vi "AIM664 VL Receive.vi"() -> ()   [LabVIEW 2020]
uses:
  AIM664LV.lvlib
panel:
  out "error out":errorcluster
  out "MsgErrorCount 2":u32
  out "MsgCount 2":u32
  out "MsgErrorCount":u32
  out "MsgCount":u32
  out "ReadBuffer 2":u8[](array[numeric])
  out "MsgRead 2":u32
  out "ReadBuffer":u8[](array[numeric])
  out "MsgRead":u32
  in  "RxModeControlIn":T1={"ReceiveMode"=1, "DefaultPayloadMode"=0, "DefaultCronoMode"=1, "GlbMonBufferSizeIn"=0, "RerosDefaultOutputPortmap"=0} {"ReceiveMode" items=["FDX_RX_CHRONO", "FDX_RX_VL"]; "DefaultPayloadMode" items=["FDX_PAYLOAD_FULL", "FDX_PAYLOAD_IP_EXT", "FDX_PAYLOAD_IP", "FDX_PAYLOAD_MAC"]; "DefaultCronoMode" items=["cFDX_RX_DEFAULT_ENA_CNT", "FDX_RX_DEFAULT_MON_ENA_ALL", "FDX_RX_DEFAULT_MON_ENA_GOOD"]}
  in  "PortMap":u32
  in  "While-Loop-Stop":bool
  in  "UdpPort2Description":T2={"PortType"=0, "UdpSrc"=2, "IpSrc"=167846145, "VlId"=10, "IpDst"=3772776458, "UdpDst"=2, "SubVlId"=0, "UdpNumBufMessages"=1, "UdpMaxMessageSize"=128, "UdpSamplingRate"=16} {"IpDst" format="%x"; "IpSrc" format="%x"; "PortType" items=["FDX_UDP_SAMPLING", "FDX_UDP_QUEUING", "FDX_UDP_RX_SAP", "FDX_UDP_TX_SAP"]}
  in  "UdpPort1Description":T2={"PortType"=0, "UdpSrc"=1, "IpSrc"=167846145, "VlId"=10, "IpDst"=3772776458, "UdpDst"=1, "SubVlId"=0, "UdpNumBufMessages"=1, "UdpMaxMessageSize"=128, "UdpSamplingRate"=32} {"IpDst" format="%x"; "IpSrc" format="%x"; "PortType" items=["FDX_UDP_SAMPLING", "FDX_UDP_QUEUING", "FDX_UDP_RX_SAP", "FDX_UDP_TX_SAP"]}
  in  "VLControl":T3={"VLId"=10, "VLRange"=1, "EnableMode"=4, "PayloadMode"=0, "TCBIndex"=0, "VerificationMode"=0, "Bag"=8, "Jitter"=1, "MaxFrameLength"=1024, "MaxSkew"=5000, "VLBufSize"=0, "FilterMode"=0, "FilterPosition"=0, "Padding"=0, "FilterMask"=0, "FilterData"=0, "MinFrameLength"=0} {"EnableMode" items=["FDX_RX_VL_DIS "=0, "FDX_RX_VL_ENA_STAT"=1, "FDX_RX_VL_ENA_CNT "=2, "FDX_RX_VL_ENA_MON_ALL"=3, "FDX_RX_VL_ENA_MON_GOOD"=7, "FDX_RX_VL_ENA_EXT"=4]; "PayloadMode" items=["FDX_PAYLOAD_FULL", "FDX_PAYLOAD_IP_EXT", "FDX_PAYLOAD_IP", "FDX_PAYLOAD_MAC"]; "VerificationMode" items=["FDX_RX_VL_CHECK_ENA_DEFAULT"=65535, "FDX_RX_VL_CHECK_REDMAM"=16, "DX_RX_VL_CHECK_TRAFIC"=8, "FDX_RX_VL_CHECK_FRAMESIZE"=4, "FDX_RX_VL_CHECK_SNINTEG"=2, "FDX_RX_VL_CHECK_INVPAC"=1, "FDX_RX_VL_CHECK_DISA"=0]; "FilterMode" items=["FDX_RX_VL_FLT_DIS", "FDX_RX_VL_FLT_ENA ", "FDX_RX_VL_FLT_ENA_INV"]}
  out "ResourceInfo 2":T4 {"PortMode" items=[" FDX_SINGLE", "FDX_REDUNDANT"]}
  out "ResourceInfo":T4 {"PortMode" items=[" FDX_SINGLE", "FDX_REDUNDANT"]}
  in  "Input Cluster":T5={"SrvName"="local", "ClHostName"="local", "ClUser"="Brett", "ClApplication"="Test", "ClApplicationVersion"="V01.00", "ResourceID"=2, "Privileges"=4294967295} {"Privileges" items=["PRIVILEGES_ADMIN"=4294967295]}
  in  "Input Cluster":T6={"SrvName"="local", "ResourceID"=1, "ResourceType"=0} {"ResourceType" items=["Board", "Port"]}
  out "Output Cluster 2":T7={"ResourceID"=1, "ResourceType"=0, "ResourceInfo"="AMC-FDX-2", "StructId"=0}
  in  "ServerRElement":u32=1
  in  "Input Cluster":T6={"SrvName"="local", "ResourceID"=2, "ResourceType"=1} {"ResourceType" items=["Board", "Port"]}
  out "Output Cluster":T7={"ResourceID"=2, "ResourceType"=1, "ResourceInfo"="Port1", "StructId"=0}
  in  "ServerRElement":u32=2
  out "NuOfResources":u32=3
  in  "SrvName":string="local"
  out "NuOfServers":u32=1
  # "ARINC 664 Receive data through a Virtual Link (VL)"
  # "Overview: Configure the board to write UDP blocks into a Port.\nRequirement: At least one AIM ARINC-664 board with installed AIM ARINC 664 BSP.\nRestrictions: None.\nInstruction:\n1. Run the VI.\n2. Verify the results in the indicators."
  # "Rx Port"
  # "FdxRxControlCvi (Stop Rx)"
  # "FdxLogoutCvi"
  # "Rx Port"
  # "Main UDP Read While-Loop"
  # "FdxInitCvi"
  # "CountServerResourcesCvi"
  # "GetServerResourcesCvi"
  # "FdxLoginCvi"
  # "FdxCmdRxPortInit"
  # "FdxCmdRxModeControl"
  # "FdxCmdVLRxControl"
  # "UDP Port Creation"
  # "FdxRxControlCvi  (Start Rx)"
  # "Input"
  # "GetServerResourcesCvi"
  # "QueryServerResourceCvi"
  # "QueryServerResourceCvi"
  # "Input"
  # "Input"
  # "Input"
  # "Input"
  # "Output"
  # "Input"
  # "Input"
  # "Input"
  # "Input"
  # "Input"
  # "Input"
  # "UDP Port 1 Read"
  # "UDP Port 2 Read"
  # "Input"
  # "Input"
  # "UDP Port 1"
  # "UDP Port 2"
  # "Input"
  # "Input"
  # "Output"
  # "Output"
  # "Output"
  # "UDP Port 1 Status"
  # "UDP Port 2 Status"
  # "Output"
  # "Output"
  # "Output"
  # "Output"
  # "Output"
  # "Output"
  # "Output"
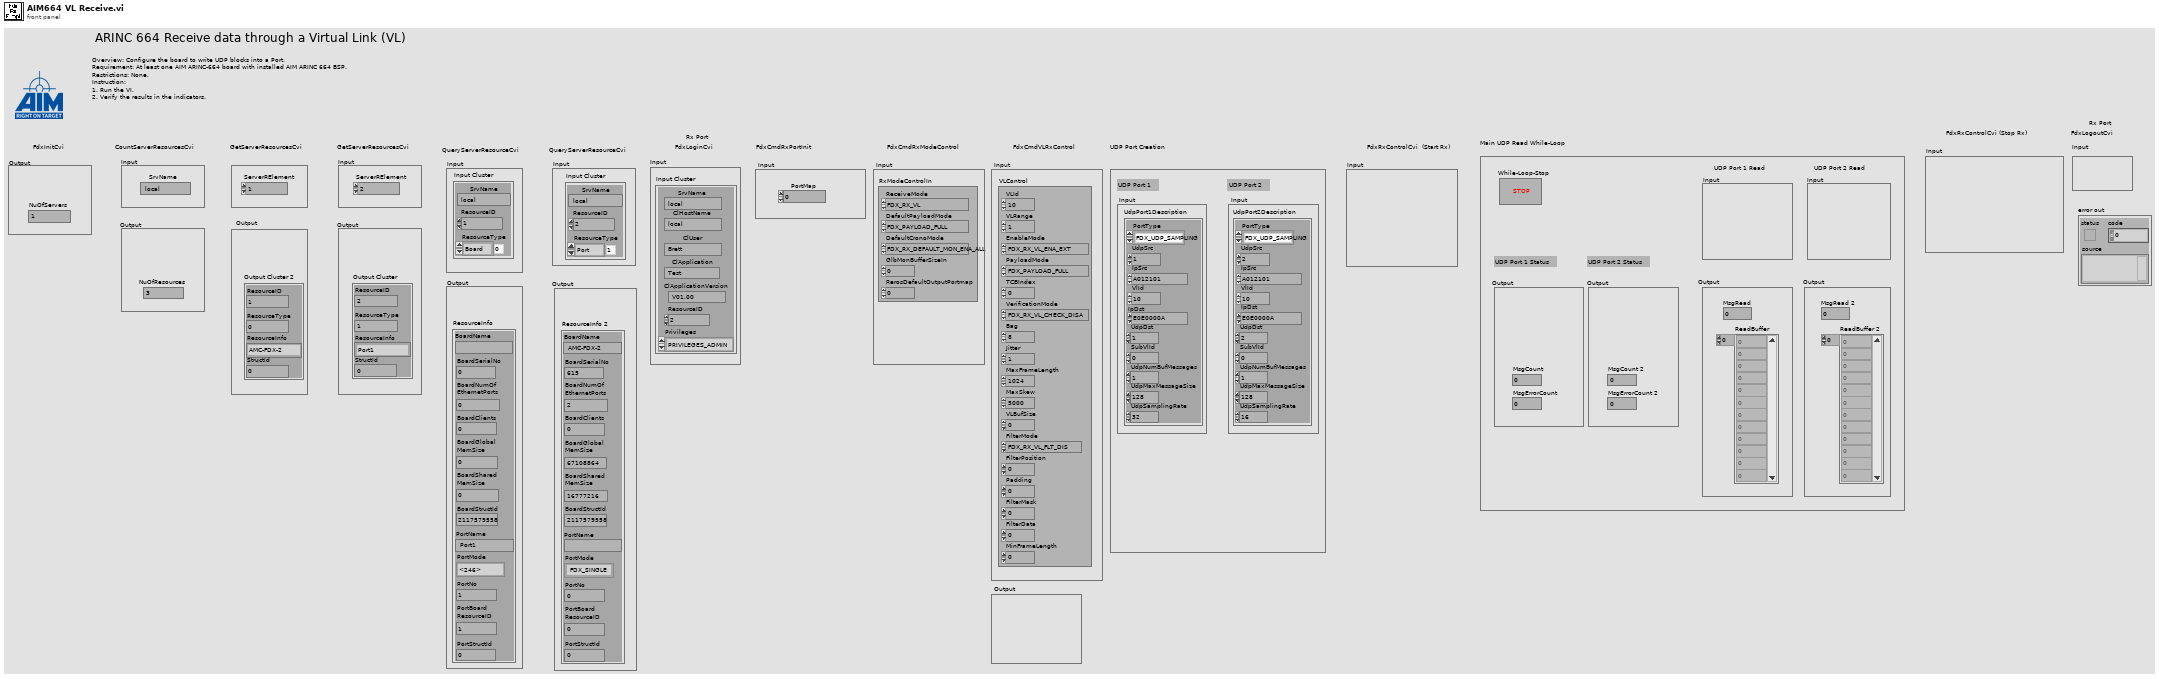
[diagram p1: front panel]
types:
  T1 = cluster{"ReceiveMode":u32, "DefaultPayloadMode":u32, "DefaultCronoMode":u32, "GlbMonBufferSizeIn":u32, "RerosDefaultOutputPortmap":u32}
  T2 = cluster{"PortType":u32, "UdpSrc":u32, "IpSrc":u32, "VlId":u32, "IpDst":u32, "UdpDst":u32, "SubVlId":u32, "UdpNumBufMessages":u32, "UdpMaxMessageSize":u32, "UdpSamplingRate":u32}
  T3 = cluster{"VLId":u32, "VLRange":u32, "EnableMode":u32, "PayloadMode":u32, "TCBIndex":u32, "VerificationMode":u32, "Bag":u32, "Jitter":u32, "MaxFrameLength":u32, "MaxSkew":u32, "VLBufSize":u32, "FilterMode":u32, "FilterPosition":u32, "Padding":u32, "FilterMask":u32, "FilterData":u32, "MinFrameLength":u32}
  T4 = cluster{"BoardName":string, "BoardSerialNo":u32, "BoardNumOf\nEthernetPorts":u32, "BoardClients":u32, "BoardGlobal\nMemSize":u32, "BoardShared\nMemSize":u32, "BoardStructId":u32, "PortName":string, "PortMode":u32, "PortNo":u32, "PortBoard\nResourceID":u32, "PortStructId":u32}
  T5 = cluster{"SrvName":string, "ClHostName":string, "ClUser":string, "ClApplication":string, "ClApplicationVersion":string, "ResourceID":u32, "Privileges":u32}
  T6 = cluster{"SrvName":string, "ResourceID":u32, "ResourceType":u32}
  T7 = cluster{"ResourceID":u32, "ResourceType":u32, "ResourceInfo":string, "StructId":u32}
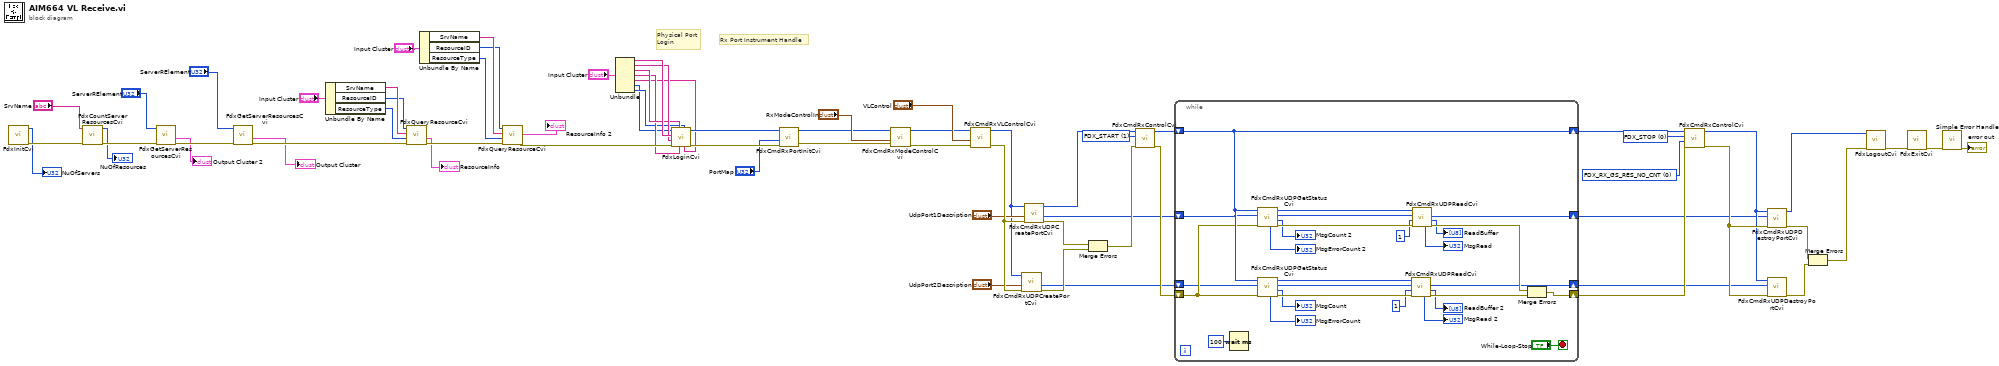
[diagram p0: block diagram]
diagram:
  w5 = u32 1 items=["FDX_STOP", "FDX_START"] ("StartMode")
  w6 = u32 0 items=["FDX_RX_GS_RES_NO_CNT", "FDX_RX_GS_RES_ALL_CNT", "FDX_RX_GS_RES_ERR_CNT "] ("GlobalStatisticReset")
  w7 = u32 0 items=["FDX_STOP", "FDX_START"] ("StartMode")
  # "Rx Port Instrument Handle"
  # "Physical Port\nLogin"
  n1 = call "FdxInitCvi.vi"() -> ("error out"=w67:errorcluster, "Number of Servers"=→"NuOfServers":u32)  [unwired: 10 in]
  n2 = call "FdxCountServerResourcesCvi.vi"("error in"=w67, "SrvName (local)"="SrvName") -> ("error out"=w66:errorcluster, "Number of Resources"=→"NuOfResources":u32)  [unwired: 8 in]
  n3 = call "FdxGetServerResourcesCvi.vi"("error in"=w66, "ServerRElement"="ServerRElement") -> ("error out"=w65:errorcluster, "ServerResourceInfo"=→"Output Cluster 2":T7)  [unwired: 4 in, 4 out]
  n4 = call "FdxGetServerResourcesCvi.vi"("error in"=w65, "ServerRElement"="ServerRElement") -> ("error out"=w68:errorcluster, "ServerResourceInfo"=→"Output Cluster":T7)  [unwired: 4 in, 4 out]
  n5 = Unbundle By Name("Input Cluster") -> ("SrvName"=w31:string, "ResourceID"=w30:u32, "ResourceType"=w29:u32)
  n6 = call "FdxQueryResourceCvi.vi"("error in"=w68, "ResourceType"=w29, "SrvName"=w31, "ResourceID"=w30) -> ("error out"=w64:errorcluster, "ResourceInfo"=→"ResourceInfo":T4)  [unwired: 5 in, 1 out]
  n7 = Unbundle By Name("Input Cluster") -> ("SrvName"=w27:string, "ResourceID"=w26:u32, "ResourceType"=w25:u32)
  n8 = call "FdxQueryResourceCvi.vi"("error in"=w64, "ResourceType"=w25, "SrvName"=w27, "ResourceID"=w26) -> ("error out"=w50:errorcluster, "ResourceInfo"=→"ResourceInfo 2":T4)  [unwired: 5 in, 1 out]
  n9 = Unbundle("Input Cluster") -> ("SrvName"=w23:string, "ClHostName"=w22:string, "ClUser"=w21:string, "ClApplication"=w20:string, "ClApplicationVersion"=w19:string, "ResourceID"=w17:u32, "Privileges"=w18:u32)
  n10 = call "FdxLoginCvi.vi"("ClApplicationVersion"=w19, "Privileges"=w18, "ClApplication"=w20, "ClUser"=w21, "error in"=w50, "ClHostName"=w22, "SrvName"=w23, "ResourceID"=w17) -> ("error out"=w53:errorcluster, "InstrumentHandle"=w37:u32)  [unwired: 2 in]
  n11 = call "FdxCmdRxPortInitCvi.vi"("error in"=w53, "PortMap"="PortMap", "InstrumentHandle_port"=w37) -> ("error out"=w54:errorcluster, "InstrumentHandle_port"=w16:u32)  [unwired: 6 in, 1 out]
  n12 = call "FdxCmdRxModeControlCvi.vi"("error in"=w54, "RxModeControlIn"="RxModeControlIn", "InstrumentHandle_port"=w16) -> ("error out"=w55:errorcluster, "InstrumentHandle_port"=w15:u32)  [unwired: 6 in, 1 out]
  n13 = call "FdxCmdRxVLControlCvi.vi"("error in"=w55, "VLControl"="VLControl", "InstrumentHandle_port"=w15) -> ("error out"=w57:errorcluster, "InstrumentHandle_port"=w14:u32)  [unwired: 7 in]
  n14 = call "FdxCmdRxUDPCreatePortCvi.vi"("error in"=w57, "UdpDescription"="UdpPort2Description", "InstrumentHandle_port"=w14) -> ("error out"=w61:errorcluster, "UdpHandle"=w38:u32)  [unwired: 6 in, 1 out]
  n15 = call "FdxCmdRxUDPCreatePortCvi.vi"("error in"=w57, "UdpDescription"="UdpPort1Description", "InstrumentHandle_port"=w14) -> ("error out"=w63:errorcluster, "UdpHandle"=w43:u32, "InstrumentHandle_port"=w13:u32)  [unwired: 6 in]
  n16 = Merge Errors(w63, w61) -> (w62:errorcluster)
  n17 = call "FdxCmdRxControlCvi.vi"("error in"=w62, "StartMode"=w5, "InstrumentHandle_port"=w13) -> ("error out"=w52:errorcluster, "InstrumentHandle_port"=w12:u32)  [unwired: 7 in]
  n18 = while {
    shift-right: [w89] -> w11
    shift-left: w12 -> [w89]
    shift-right: [w70] -> w4
    shift-left: w43 -> [w85]
    shift-right: [w74] -> w3
    shift-left: w38 -> [w84]
    shift-right: [w87] -> w8
    shift-left: w52 -> [w88]
    stop <- "While-Loop-Stop" stop-if-true
    n19 = Wait (ms)(milliseconds to wait=u32 100 ("Zu wartende ms")) -> ()  [unwired: 1 out]
    n20 = call "FdxCmdRxUDPGetStatusCvi.vi"("error in"=w88, "UdpHandle"=w85, "InstrumentHandle_port"=w89) -> ("error out"=w95:errorcluster, "MsgCount"=→"MsgCount 2":u32, "UdpHandle Out"=w72:u32, "InstrumentHandle_port"=w69:u32, "MsgErrorCount"=→"MsgErrorCount 2":u32)  [unwired: 4 in]
    n21 = call "FdxCmdRxUDPGetStatusCvi.vi"("error in"=w88, "UdpHandle"=w84, "InstrumentHandle_port"=w89) -> ("error out"=w94:errorcluster, "MsgCount"=→"MsgCount":u32, "UdpHandle Out"=w76:u32, "InstrumentHandle_port"=w73:u32, "MsgErrorCount"=→"MsgErrorCount":u32)  [unwired: 4 in]
    n22 = call "FdxCmdRxUDPReadCvi.vi"("error in"=w94, "MsgCount"=u32 1, "UdpHandle"=w76, "InstrumentHandle_port"=w73) -> ("error out"=w93:errorcluster, "ReadBuffer"=→"ReadBuffer 2":u8[], "UdpHandle  Out"=w74:u32, "MsgRead"=→"MsgRead 2":u32)  [unwired: 3 in, 1 out]
    n23 = call "FdxCmdRxUDPReadCvi.vi"("error in"=w95, "MsgCount"=u32 1, "UdpHandle"=w72, "InstrumentHandle_port"=w69) -> ("error out"=w92:errorcluster, "ReadBuffer"=→"ReadBuffer":u8[], "UdpHandle  Out"=w70:u32, "MsgRead"=→"MsgRead":u32)  [unwired: 3 in, 1 out]
    n24 = Merge Errors(w92, w93) -> (w87:errorcluster)
  }
  n25 = call "FdxCmdRxControlCvi.vi"("error in"=w8, "GlobalStatisticReset"=w6, "StartMode"=w7, "InstrumentHandle_port"=w11) -> ("error out"=w60:errorcluster, "InstrumentHandle_port"=w10:u32)  [unwired: 6 in]
  n26 = call "FdxCmdRxUDPDestroyPortCvi.vi"("error in"=w60, "UdpHandle"=w4, "InstrumentHandle_port"=w10) -> ("error out"=w59:errorcluster, "InstrumentHandle_port"=w9:u32)  [unwired: 7 in]
  n27 = call "FdxCmdRxUDPDestroyPortCvi.vi"("error in"=w60, "UdpHandle"=w3, "InstrumentHandle_port"=w10) -> ("error out"=w58:errorcluster)  [unwired: 7 in, 1 out]
  n28 = Merge Errors(w59, w58) -> (w56:errorcluster)
  n29 = call "FdxLogoutCvi.vi"("error in"=w56, "InstrumentHandle"=w9) -> ("error out"=w51:errorcluster)  [unwired: 9 in]
  n30 = call "FdxExitCvi.vi"("error in"=w51) -> ("error out"=w2:errorcluster)  [unwired: 10 in]
  n31 = call <vilib>:"Simple Error Handler.vi"("error in (no error)"=w2) -> ("error out"=→"error out":errorcluster)  [unwired: 4 in, 4 out]
